vi "Finish Stream.vi"(8 "error in (no error)":errorcluster, 11 "Orca-Flash 4.0 V2 in":refnum<class "Hamamatsu Camera.lvclass">) -> (0 "error out":errorcluster, 3 "Orca-Flash 4.0 V2 out":refnum<class "Hamamatsu Camera.lvclass">)   [LabVIEW 2018, in "Hamamatsu Camera.lvlib" / "Hamamatsu Camera.lvclass"]
uses:
  Hamamatsu Camera.lvclass
  C:/FlashGordon/Development/Hardware/Camera/Camera.lvclass
  Resources/GLOBAL/GLOBAL Time-critical.vi
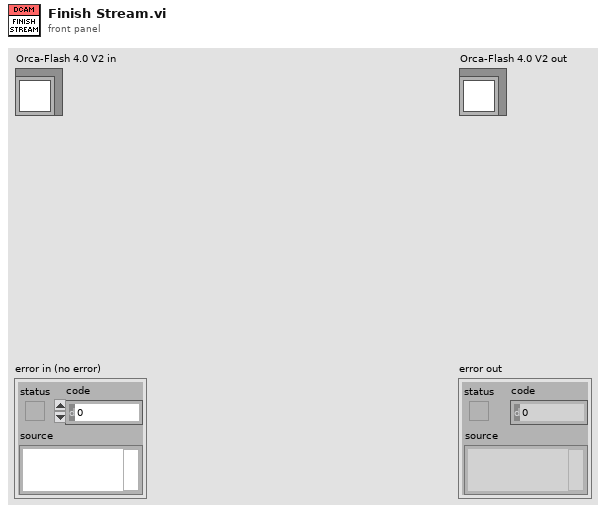
[diagram p1: front panel]
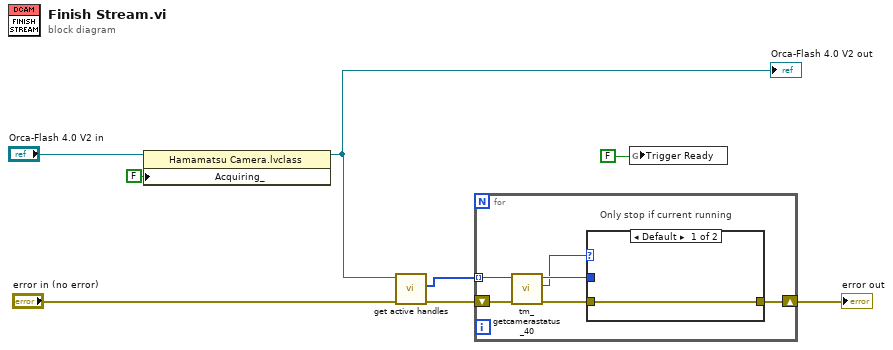
[diagram p0: block diagram]
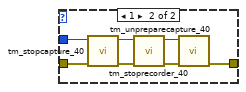
[diagram p2: hidden frame]
diagram:
  n1 = property class="Hamamatsu Camera.lvclass"(reference="Orca-Flash 4.0 V2 in", "Acquiring_"=FALSE ("Live Mode")) -> (reference out=w1:refnum<class "Hamamatsu Camera.lvclass">)  [unwired: 1 in, 1 out]
  "Orca-Flash 4.0 V2 out" <- w1
  n2 = call-dynamic "get active handles.vi"("error in (no error)"="error in (no error)", "Hamamatsu Camera in"=w1) -> ("error out"=w3:errorcluster, "Handles"=w2:u32[])  [unwired: 5 in, 3 out]
  n3 = for {
    tunnel: w2 -> [w10] mode=indexing
    shift-right: [w14] -> w6
    shift-left: w3 -> [w13]
    # "Only stop if current running"
    n4 = call <userlib>:"tm_getcamerastatus_40.vi"("error in (no error)"=w13, "Handle in"=w10) -> ("error out"=w12:errorcluster, "Status"=w9:i32, "Handle out"=w11:u32)  [unwired: 7 in]
    n5 = case shown="Default" w9 {
      tunnel: w12 -> [w15 w22]
      tunnel: w11 -> [_ w21]
      tunnel: [w15 w16] -> w14
      frame Default {
      }
      frame 1 {
        n6 = call <userlib>:"tm_stopcapture_40.vi"("error in (no error)"=w22, "Handle in"=w21) -> ("error out"=w20:errorcluster, "Handle out"=w19:u32)  [unwired: 8 in]
        n7 = call <userlib>:"tm_stoprecorder_40.vi"("error in (no error)"=w20, "Handle in"=w19) -> ("error out"=w17:errorcluster, "Handle out"=w18:u32)  [unwired: 8 in]
        n8 = call <userlib>:"tm_unpreparecapture_40.vi"("error in (no error)"=w17, "Handle in"=w18) -> ("error out"=w16:errorcluster)  [unwired: 8 in, 1 out]
      }
    }
  }
  "error out" <- w6
  n9 = global write "GLOBAL Time-critical.vi" "Trigger Ready"(FALSE ("new element/subarray")) -> ()
